vi "TestWrites.vi"() -> ()   [LabVIEW 2017]
uses:
  Global 1.vi
panel:
  out "Indicator":dbl
  out "Time per write":dbl[](array[numeric])
  in  "Iterations":i32=5000
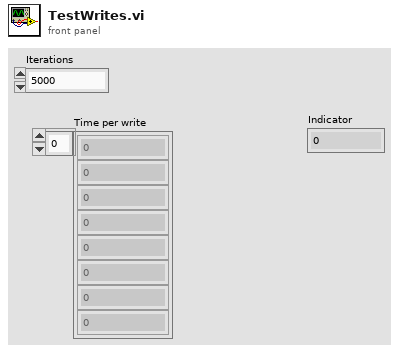
[diagram p1: front panel]
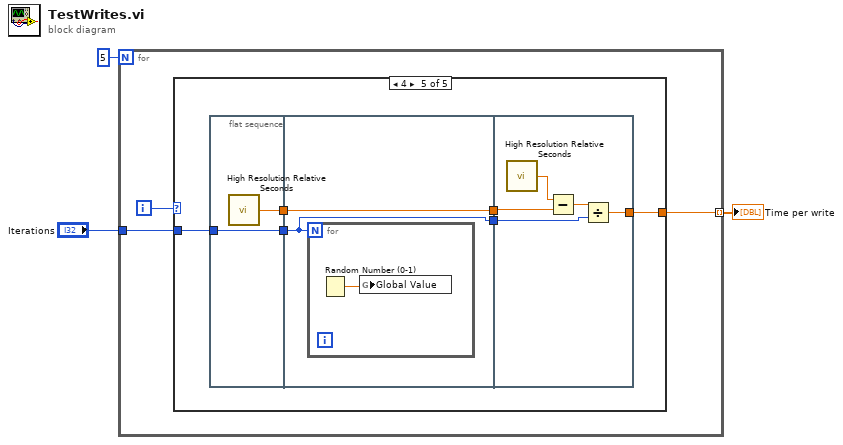
[diagram p0: block diagram]
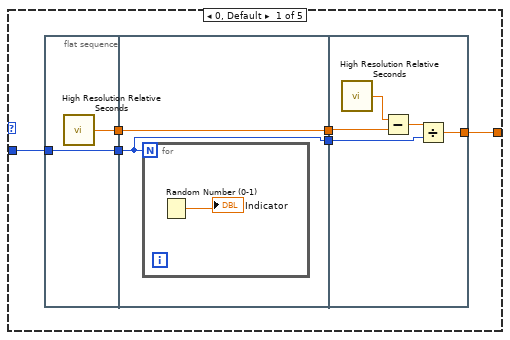
[diagram p2: hidden frame]
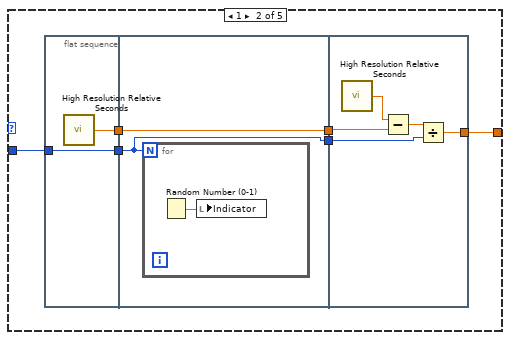
[diagram p3: hidden frame]
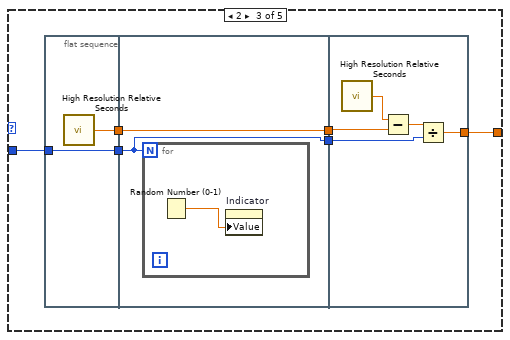
[diagram p4: hidden frame]
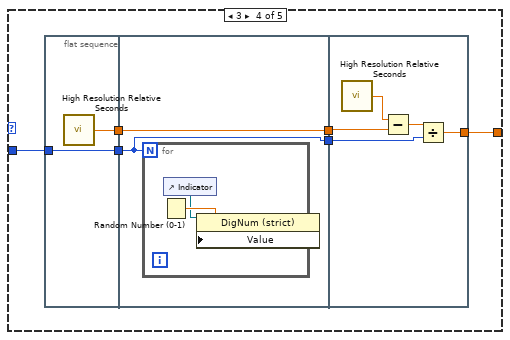
[diagram p5: hidden frame]
diagram:
  n1 = for {
    N: 5 -> [_]
    tunnel: "Iterations" -> [w5]
    tunnel: [w4] -> w2 mode=indexing
    i -> [w6]
    n2 = case shown="4" w6 {
      tunnel: w5 -> [w10 w26 w42 w58 w75]
      tunnel: [w7 w23 w39 w55 w72] -> w4
      frame 0, Default {
        n3 = flat-sequence {
          tunnel: [w14] -> w11
          tunnel: w10 -> [w13]
          tunnel: [w13] -> w9
          tunnel: [w16] -> w12
          tunnel: w11 -> [w16]
          tunnel: w9 -> [w15]
          tunnel: [w15] -> w8
          tunnel: w12 -> [w21]
          tunnel: w8 -> [w19]
          tunnel: [w18] -> w7
          frame #0 {
            n4 = call <vilib>:"High Resolution Relative Seconds.vi"() -> ("relative seconds"=w14:dbl)
          }
          frame #1 {
            n5 = for {
              N: w15 -> [_]
              n6 = Random Number (0-1)() -> (number: 0 to 1=→"Indicator":dbl)
            }
          }
          frame #2 {
            n7 = call <vilib>:"High Resolution Relative Seconds.vi"() -> ("relative seconds"=w22:dbl)
            n8 = Subtract(x=w22, y=w21) -> (x-y=w20:dbl)
            n9 = Divide(x=w20, y=w19) -> (x/y=w18:dbl)
          }
        }
      }
      frame 1 {
        n10 = flat-sequence {
          tunnel: [w30] -> w27
          tunnel: w26 -> [w29]
          tunnel: [w29] -> w25
          tunnel: [w32] -> w28
          tunnel: w27 -> [w32]
          tunnel: w25 -> [w31]
          tunnel: [w31] -> w24
          tunnel: w28 -> [w37]
          tunnel: w24 -> [w35]
          tunnel: [w34] -> w23
          frame #0 {
            n11 = call <vilib>:"High Resolution Relative Seconds.vi"() -> ("relative seconds"=w30:dbl)
          }
          frame #1 {
            n12 = for {
              N: w31 -> [_]
              n13 = Random Number (0-1)() -> (number: 0 to 1=w33:dbl)
              n14 = local write "Indicator"(w33) -> ()
            }
          }
          frame #2 {
            n15 = call <vilib>:"High Resolution Relative Seconds.vi"() -> ("relative seconds"=w38:dbl)
            n16 = Subtract(x=w38, y=w37) -> (x-y=w36:dbl)
            n17 = Divide(x=w36, y=w35) -> (x/y=w34:dbl)
          }
        }
      }
      frame 2 {
        n18 = flat-sequence {
          tunnel: [w46] -> w43
          tunnel: w42 -> [w45]
          tunnel: [w45] -> w41
          tunnel: [w48] -> w44
          tunnel: w43 -> [w48]
          tunnel: w41 -> [w47]
          tunnel: [w47] -> w40
          tunnel: w44 -> [w53]
          tunnel: w40 -> [w51]
          tunnel: [w50] -> w39
          frame #0 {
            n19 = call <vilib>:"High Resolution Relative Seconds.vi"() -> ("relative seconds"=w46:dbl)
          }
          frame #1 {
            n20 = for {
              N: w47 -> [_]
              n21 = Random Number (0-1)() -> (number: 0 to 1=w49:dbl)
              n22 = property on="Indicator" class="DigNum (strict)"("Value"=w49) -> ()  [unwired: 2 in, 2 out]
            }
          }
          frame #2 {
            n23 = call <vilib>:"High Resolution Relative Seconds.vi"() -> ("relative seconds"=w54:dbl)
            n24 = Subtract(x=w54, y=w53) -> (x-y=w52:dbl)
            n25 = Divide(x=w52, y=w51) -> (x/y=w50:dbl)
          }
        }
      }
      frame 3 {
        n26 = flat-sequence {
          tunnel: [w62] -> w59
          tunnel: w58 -> [w61]
          tunnel: [w61] -> w57
          tunnel: [w64] -> w60
          tunnel: w59 -> [w64]
          tunnel: w57 -> [w63]
          tunnel: [w63] -> w56
          tunnel: w60 -> [w70]
          tunnel: w56 -> [w68]
          tunnel: [w67] -> w55
          frame #0 {
            n27 = call <vilib>:"High Resolution Relative Seconds.vi"() -> ("relative seconds"=w62:dbl)
          }
          frame #1 {
            n28 = for {
              N: w63 -> [_]
              n29 = Random Number (0-1)() -> (number: 0 to 1=w66:dbl)
              n30 = control-ref of="Indicator"() -> (w65:refnum<vi>)
              n31 = property on="Property Node" class="DigNum (strict)"(reference=w65, "Value"=w66) -> ()  [unwired: 1 in, 2 out]
            }
          }
          frame #2 {
            n32 = call <vilib>:"High Resolution Relative Seconds.vi"() -> ("relative seconds"=w71:dbl)
            n33 = Subtract(x=w71, y=w70) -> (x-y=w69:dbl)
            n34 = Divide(x=w69, y=w68) -> (x/y=w67:dbl)
          }
        }
      }
      frame 4 {
        n35 = flat-sequence {
          tunnel: [w79] -> w76
          tunnel: w75 -> [w78]
          tunnel: [w78] -> w74
          tunnel: [w81] -> w77
          tunnel: w76 -> [w81]
          tunnel: w74 -> [w80]
          tunnel: [w80] -> w73
          tunnel: w77 -> [w86]
          tunnel: w73 -> [w84]
          tunnel: [w83] -> w72
          frame #0 {
            n36 = call <vilib>:"High Resolution Relative Seconds.vi"() -> ("relative seconds"=w79:dbl)
          }
          frame #1 {
            n37 = for {
              N: w80 -> [_]
              n38 = Random Number (0-1)() -> (number: 0 to 1=w82:dbl)
              n39 = global write "Global 1.vi" "Global Value"(w82) -> ()
            }
          }
          frame #2 {
            n40 = call <vilib>:"High Resolution Relative Seconds.vi"() -> ("relative seconds"=w87:dbl)
            n41 = Subtract(x=w87, y=w86) -> (x-y=w85:dbl)
            n42 = Divide(x=w85, y=w84) -> (x/y=w83:dbl)
          }
        }
      }
    }
  }
  "Time per write" <- w2
